vi "g_RobotSettingsALB.vi"(7 "Action":enum16{"read", "write"}(ring), 10 "Settings":T1) -> (2 "Settings out":T1)   [LabVIEW 2017]
uses:
  CtrlRefs/SettingsALB.ctl
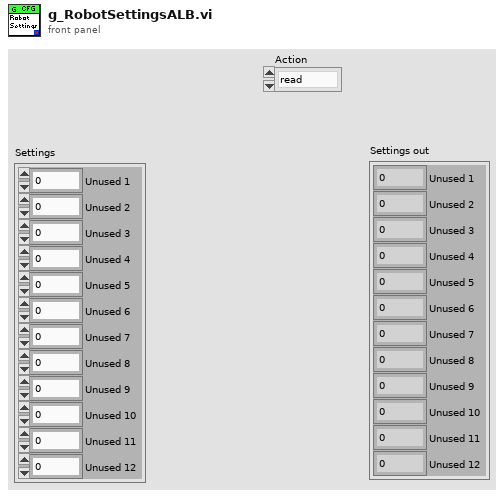
[diagram p1: front panel]
types:
  T1 = typedef "SettingsALB.ctl" = cluster{"Unused 1":dbl, "Unused 2":dbl, "Unused 3":dbl, "Unused 4":dbl, "Unused 5":dbl, "Unused 6":dbl, "Unused 7":dbl, "Unused 8":dbl, "Unused 9":dbl, "Unused 10":dbl, "Unused 11":dbl, "Unused 12":dbl}
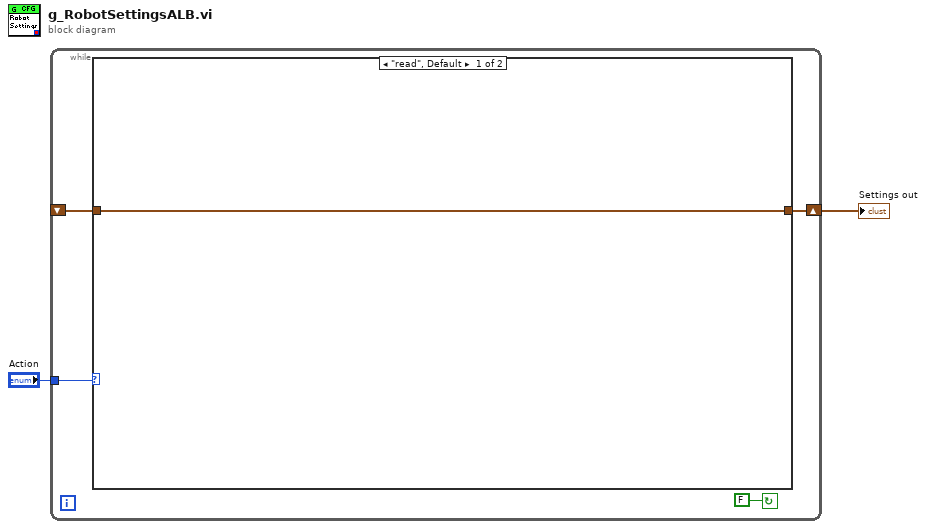
[diagram p0: block diagram]
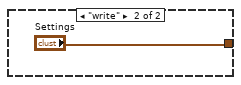
[diagram p2: hidden frame]
diagram:
  n1 = while {
    tunnel: "Action" -> [w5]
    shift-right: [w4] -> w1
    shift-left: _ -> [w3]
    stop <- FALSE continue-if-true
    n2 = case shown="\"read\", Default" w5 {
      tunnel: [w7 "Settings"] -> w4
      tunnel: w3 -> [w7 _]
      frame "read", Default {
      }
      frame "write" {
      }
    }
  }
  "Settings out" <- w1
